vi "mergeVISAPropNode.vi"   [LabVIEW 2018]
doc: "获取（读取）和/或设置（写入）引用的属性。 该节点的操作与属性节点的操作相同。"
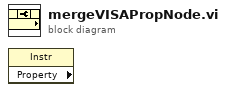
[diagram p0: block diagram]
diagram:
  n1 = property class="Instr" props=[]() -> ()  [unwired: 2 in, 3 out]
